vi "isNumber.vi"(8 "error in (no error)":errorcluster, 10 "string":string, 11 "CommandParser in":refnum<class "CommandParser.lvclass">) -> (0 "error out":errorcluster, 2 "isNumber?":bool, 3 "CommandParser out":refnum<class "CommandParser.lvclass">)   [LabVIEW 2020, in "CommandParser.lvclass"]
uses:
  CommandParser.lvclass
  <vilib>/regexp/Match Regular Expression.xnode
panel:
  out "after match":string
  out "whole match":string
  out "before match":string
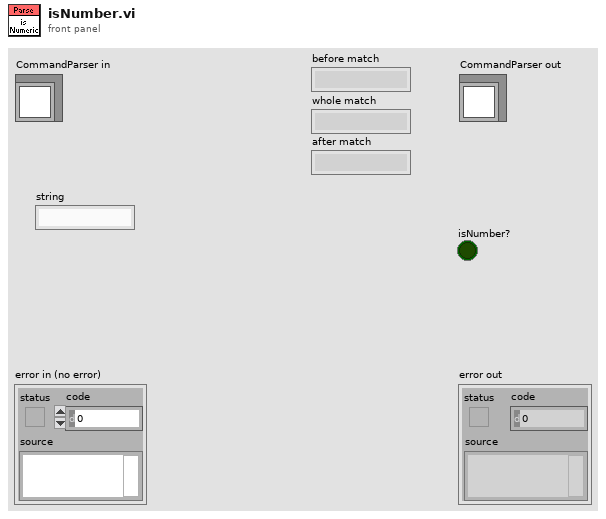
[diagram p1: front panel]
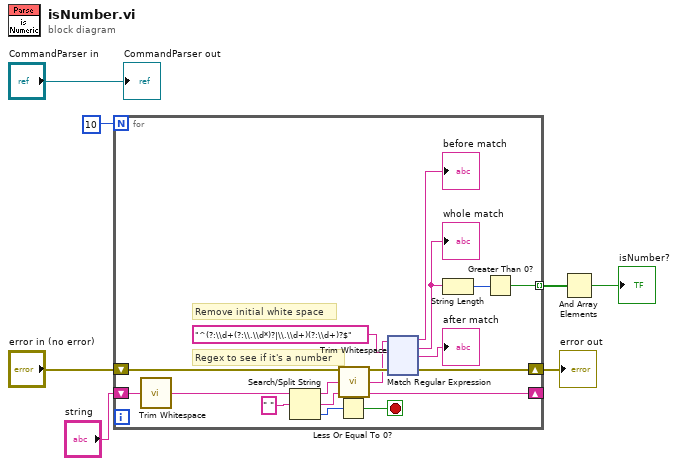
[diagram p0: block diagram]
diagram:
  n1 = for {
    N: 10 -> [_]
    tunnel: [w16] -> w1 mode=indexing
    shift-right: [w21] -> w5
    shift-left: "error in (no error)" -> [w22]
    shift-right: [w12] -> _
    shift-left: "string" -> [w9]
    stop <- w11 stop-if-true
    # "Regex to see if it's a number"
    # "Remove initial white space"
    n2 = call <vilib>:"Trim Whitespace.vi"("string"=w9) -> ("trimmed string"=w8:string)  [unwired: 1 in]
    n3 = Search/Split String(string=w8, search string/char (-)=" ") -> (substring before match=w13:string, match + rest of string=w12:string, offset of match=w10:i32)  [unwired: 1 in]
    n4 = Less Or Equal To 0?(x=w10) -> (x <= 0?=w11:bool)
    n5 = call <vilib>:"Trim Whitespace.vi"("string"=w13) -> ("trimmed string"=w15:string)  [unwired: 1 in]
    n6 = xnode "Match Regular Expression"("input string"=w15, "regular expression"="^(?:\\d+(?:\\.\\d*)?|\\.\\d+)(?:\\d+)?$", "error in"=w22) -> ("before match"=→"before match":string, "whole match"=w18:string, "after match"=→"after match":string, "error out"=w21:errorcluster)  [unwired: 3 in, 1 out]
    "whole match" <- w18
    n7 = String Length(string=w18) -> (length=w17:i32)
    n8 = Greater Than 0?(x=w17) -> (x > 0?=w16:bool)
  }
  "error out" <- w5
  n9 = And Array Elements(Boolean array=w1) -> (logical AND=→"isNumber?":bool)
  "CommandParser out" <- "CommandParser in"
